vi "错误-配置项未处理.vi"(7 "段名":string, 8 "error out":errorcluster={"status"=TRUE, "code"=0, "source"=""}, 11 "键名":string) -> (0 "输出簇":errorcluster)   [LabVIEW 2017]
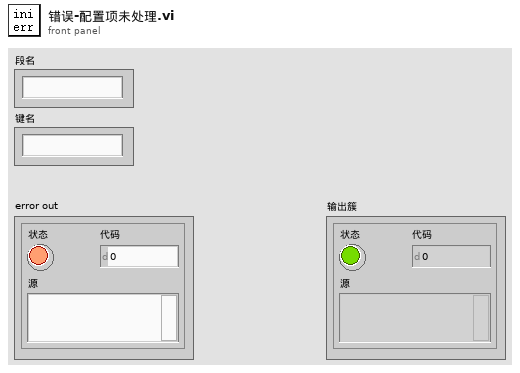
[diagram p1: front panel]
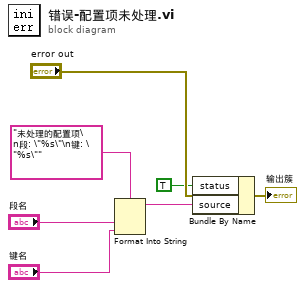
[diagram p0: block diagram]
diagram:
  n1 = Format Into String(format string="未处理的配置项\n段: \"%s\"\n键: \"%s\"" ("格式字符串"), "段名", "键名") -> (resulting string=w4:string)  [unwired: 2 in, 1 out]
  n2 = Bundle By Name(cluster="error out", "status"=TRUE, "source"=w4) -> (→"输出簇":errorcluster)
